vi "WhileLoop.vi"() -> ()   [LabVIEW 2020]
panel:
  in  "Boolean":bool
  out "x+y":i32
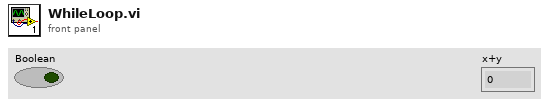
[diagram p1: front panel]
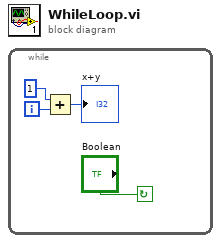
[diagram p0: block diagram]
diagram:
  n1 = while {
    i -> [w4]
    stop <- "Boolean" continue-if-true
    n2 = Add(x=1, y=w4) -> (x+y=→"x+y":i32)
  }
